vi "inHg_to_hPa.vi"(1 "inHg":sgl) -> (0 "hPa":sgl)   [LabVIEW 2012]
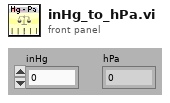
[diagram p1: front panel]
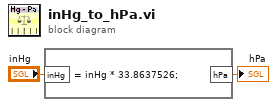
[diagram p0: block diagram]
diagram:
  n1 = formula code="hPa = inHg * 33.8637526;"("inHg"="inHg") -> ("hPa"=→"hPa":dbl)
